vi "TW Edit - Stage 1.vi"(6 "Debug":bool, 8 "error in":errorcluster) -> (0 "error out":errorcluster, 4 "Result for debugging":cluster{"Name":string, picture[]}[](array[cluster]))   [LabVIEW 2021, in "Plugin Generator.lvlib"]
uses:
  Plugin Generator.lvlib
  Typedef/Plugin OS.ctl
  <vilib>/Utility/EditLVLibs/Rename And Move Entire Library By Name.vi
  <vilib>/Utility/EditLVLibs/Rename And Move Entire Library By Path.vi
  <vilib>/Utility/EditLVProj/Edit LVProj.lvlib
panel:
  in  "Text color":u32(colorbox)
  in  "Background":u32(colorbox)=7208704
  in  "Name":string
  in  "Plugin OS":T1=enum."Env Server" caption="OS"
  in  "Project Name":string
  in  "User Project Path":path
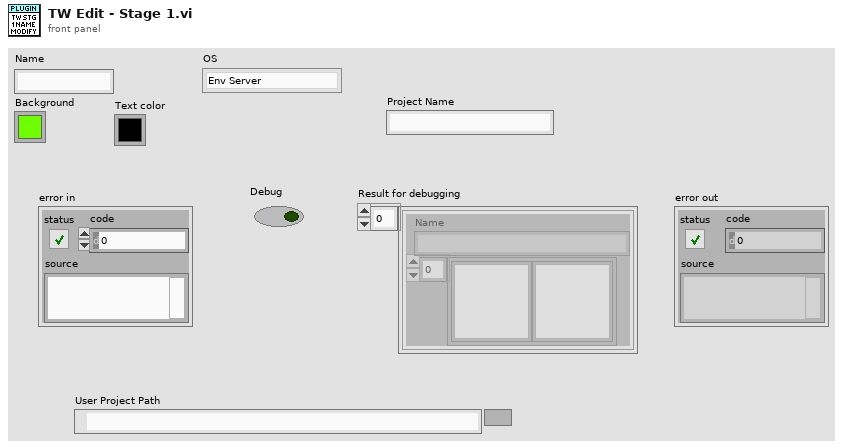
[diagram p1: front panel]
types:
  T1 = typedef "Plugin Generator.lvlib/Plugin OS.ctl" = enum16{"Linux RT", "Env Server"}
  T2 = typedef "Edit LVProj.lvlib/Library And VI References.ctl" = cluster{"Target Reference":refnum<vi>, "VI References":refnum<vi>[], "Library References":refnum<vi>[]}
  T3 = enum16{"open", "replace", "create", "open or create", "replace or create", "replace or create with confirmation"}
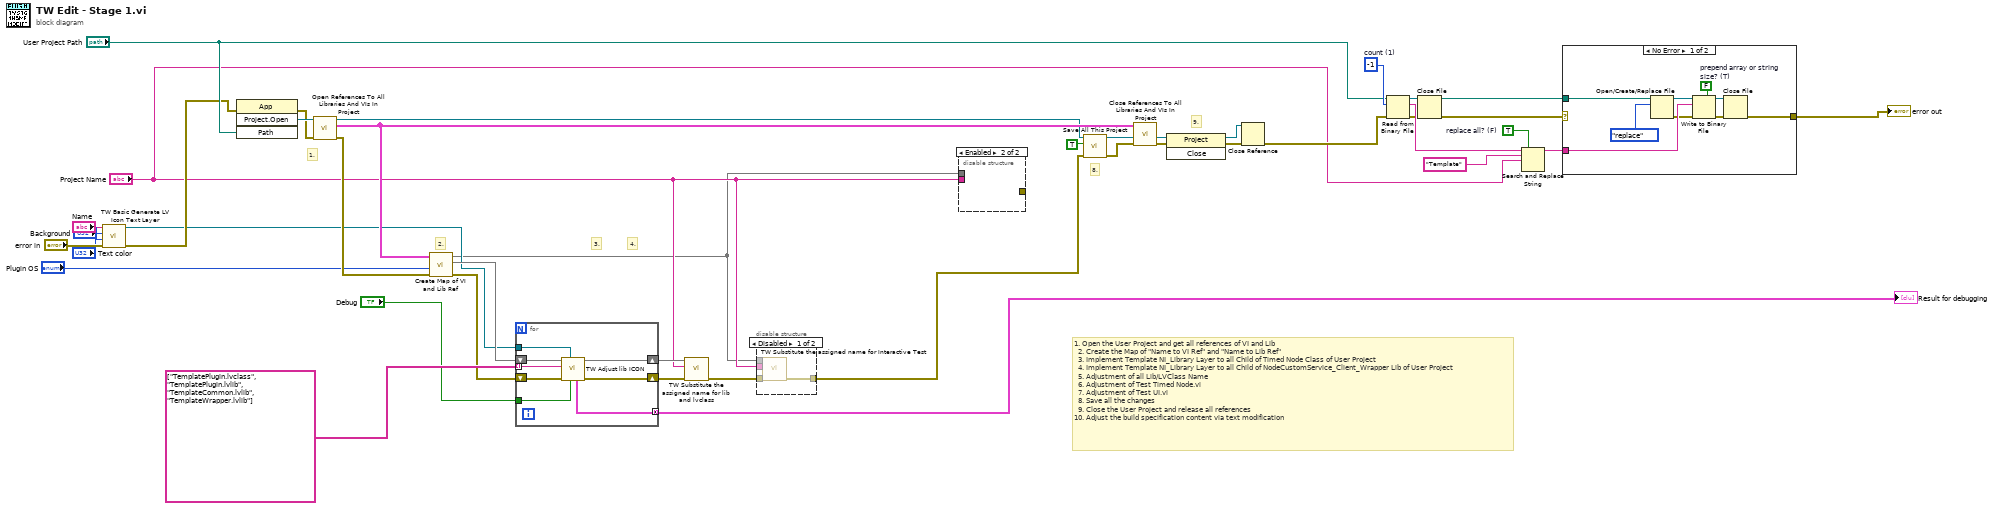
[diagram p0: block diagram]
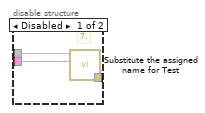
[diagram p3: hidden frame]
diagram:
  w25 = TRUE  # replace all? (F)
  w28 = -1  # count (1)
  # "9."
  # "2."
  # "8."
  # "4."
  # "3."
  # "1."
  # "1. Open the User Project and get all references of VI and Lib\n  2. Create the Map of \"Name to VI Ref\" and \"Name to Lib Ref\"\n  3. Implement Template NI_Library Layer to all Child of Timed Node Class of User Project\n  4. Implement Template NI_Library Layer to all Child of NodeCustomService_Client_Wrapper Lib of User Project\n  5. Adjustment of all Lib/LVClass Name\n  6. Adjustment of Test Timed Node.vi\n  7. Adjustment of Test UI.vi\n  8. Save all the changes\n  9. Close the User Project and release all references\n10. Adjust the build specification content via text modification"
  n1 = call "TW Basic Generate LV Icon Text Layer.vi"("error in (no error)"="error in", "Text color"="Text color", "Background"="Background", "Name"="Name") -> ("error out"=w16:errorcluster, "Icon.lvlclass out"=w10:refnum<class "Icon.lvclass">)  [unwired: 5 in, 1 out]
  n2 = invoke class="App" method="Project.Open"(error in=w16, "Path"="User Project Path") -> (error out=w31:errorcluster, "Project:Open"=w36:refnum<vi>)  [unwired: 2 in, 2 out]
  n3 = call <vilib>:"Open References To All Libraries And VIs In Project.vi"("error in (no error)"=w31, "Project in"=w36) -> ("error out"=w30:errorcluster, "VI and Library References"=w40:T2[], "Project out"=w38:refnum<vi>)  [unwired: 7 in]
  n4 = call "Create Map of VI and Lib Ref.vi"("error in"=w30, "Plugin OS"="Plugin OS", "VI and Library References"=w40) -> ("error out"=w9:errorcluster, "Map - LibRef"=w11:map{string, refnum<vi>}, "Map - VIRef"=w1:map{string, refnum<vi>})  [unwired: 6 in]
  n5 = for {
    tunnel: string[] ["TemplatePlugin.lvclass", "TemplatePlugin.lvlib", "TemplateCommon.lvlib", "TemplateWrapper.lvlib"] -> [w49] mode=indexing
    shift-right: [w47] -> w7
    shift-left: w11 -> [w48]
    tunnel: w10 -> [w46]
    tunnel: [w45] -> w5 mode=concatenating
    shift-right: [w43] -> w6
    shift-left: w9 -> [w44]
    tunnel: "Debug" -> [w42]
    n6 = call "TW Adjust lib ICON.vi"("Debug"=w42, "Overlay Icon"=w46, "error in"=w44, "Library Name"=w49, "Name to Lib Map"=w48) -> ("error out"=w43:errorcluster, "Name to Lib Map out"=w47:map{string, refnum<vi>}, "Result for debugging"=w45:cluster{"Name":string, picture[]}[])  [unwired: 4 in]
  }
  "Result for debugging" <- w5
  n7 = call "TW Substitute the assigned name for lib and lvclass.vi"("error in"=w6, "Project Name"="Project Name", "Name to Lib Map"=w7) -> ("error out"=w4:errorcluster)  [unwired: 7 in, 1 out]
  n8 = disable-structure shown="Disabled" {
    disable-tunnel: w4 -> [w53 w54]
    disable-tunnel: [w52 w54] -> w3
    disable-tunnel: "Project Name" -> [w51 _]
    disable-tunnel: w1 -> [w50 _]
    frame Disabled {
      n9 = call "TW Substitute the assigned name for Interactive Test.vi"("error in"=w53, "Project Name"=w51, "Name to VI Map"=w50) -> ("error out"=w52:errorcluster)  [unwired: 8 in]
    }
    frame Enabled {
    }
  }
  n10 = disable-structure shown="Enabled" {
    disable-tunnel: [w57 _] -> _
    disable-tunnel: w1 -> [w56 _]
    disable-tunnel: "Project Name" -> [w55 _]
    frame Disabled {
      # "7."
      n11 = call "Substitute the assigned name for Test.vi"("Project Name"=w55, "Name to VI Map"=w56) -> ("error out"=w57:errorcluster)  [unwired: 9 in]
    }
    frame Enabled {
    }
  }
  n12 = call <vilib>:"Save All This Project.vi"("error in (no error)"=w3, "Exclude Dependencies? (F)"=TRUE, "Project in"=w38) -> ("error out"=w37:errorcluster, "Project out"=w33:refnum<vi>)  [unwired: 7 in]
  n13 = call <vilib>:"Close References To All Libraries And VIs In Project.vi"("error in (no error)"=w37, "VI and Library References"=w40) -> ("error out"=w32:errorcluster)  [unwired: 9 in]
  n14 = invoke class="Project" method="Close"(reference=w33, error in=w32) -> (reference out=w34:refnum<vi>, error out=w35:errorcluster)  [unwired: 1 in, 1 out]
  n15 = Close Reference(reference=w34, error in (no error)=w35) -> (error out=w19:errorcluster)
  n16 = Read from Binary File(8:w19, 10:w28, 11:"User Project Path") -> (0:w24:errorcluster, 2:w27:string, 3:w23:refnum<file>)  [unwired: 3 in, 1 out]
  n17 = Close File(refnum=w23, error in=w24) -> (path=w21:path, error out=w20:errorcluster)
  n18 = Search and Replace String(replace all?=w25, input string=w27, search string="Template", replace string="Project Name") -> (result string=w22:string)  [unwired: 4 in, 3 out]
  n19 = case shown="No Error" w20 {
    selector: w20 -> [_ w67]
    tunnel: w22 -> [w64 _]
    tunnel: [w63 w67] -> w41
    tunnel: w21 -> [w61 _]
    frame No Error {
      w58 = FALSE  # prepend array or string size? (T)
      n20 = Open/Create/Replace File(file path (use dialog)=w61, operation (0:open)=T3."replace") -> (refnum out=w59:refnum<file>, error out=w62:errorcluster)  [unwired: 4 in, 1 out]
      n21 = Write to Binary File(file (use dialog)=w59, data=w64, error in=w62, 5:w58) -> (refnum out=w66:refnum<file>, error out=w65:errorcluster)  [unwired: 2 in, 1 out]
      n22 = Close File(refnum=w66, error in=w65) -> (error out=w63:errorcluster)  [unwired: 1 out]
    }
    frame Error {
    }
  }
  "error out" <- w41
